vi "CSM - List Status in Broadcast Registry.vi"(8 "error in (no error)":errorcluster) -> (0 "error out":errorcluster, 3 "Status in Registry":string[](array[string]))   [LabVIEW 2020, in "Communicable State Machine.lvlib"]
uses:
  Communicable State Machine.lvlib
  Operation-BroadcastRegistry.ctl
  global-Broadcast Cache Change Flag.vi
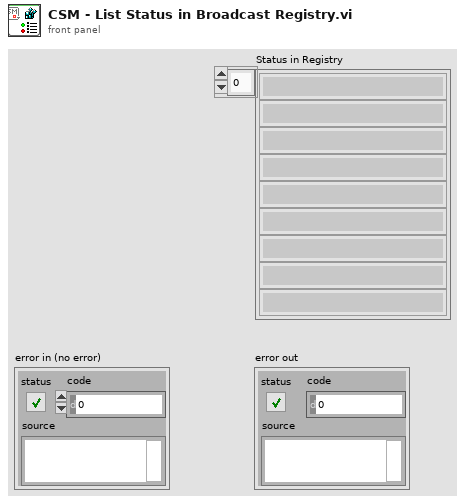
[diagram p1: front panel]
types:
  T1 = typedef "Communicable State Machine.lvlib/Operation-BroadcastRegistry.ctl" = enum16{"Delete Source Module", "Delete Target Module", "Remove Module", "Register", "Unregister", "Check", "List Status", "List Entries"}
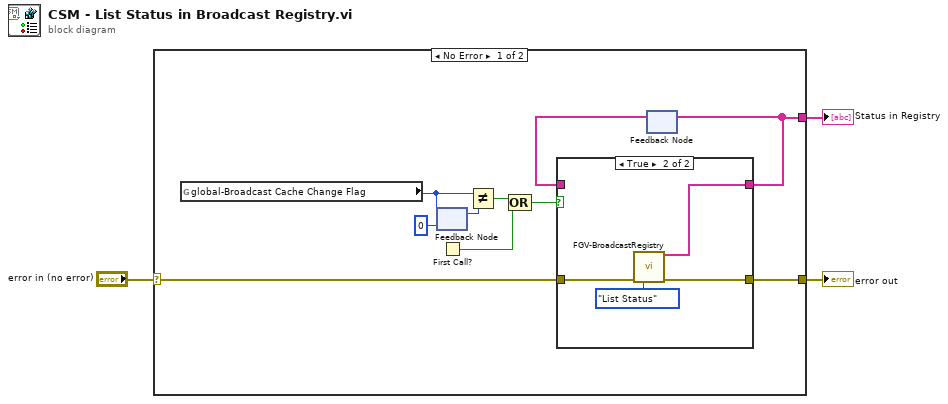
[diagram p0: block diagram]
diagram:
  n1 = case shown="No Error" "error in (no error)" {
    selector: "error in (no error)" -> [w13 w20]
    tunnel: [w6 _] -> w2
    tunnel: [w4 w20] -> w1
    frame No Error {
      n2 = global read "global-Broadcast Cache Change Flag.vi" "global-Broadcast Cache Change Flag"() -> (w10:u64)
      n3 = feedback #1(u64 0 ("global-Broadcast Cache Change Flag")) -> (w11:u64)
      n4 = feedback-in #1(w10) -> ()
      n5 = First Call?() -> (First Call?: T/F=w9:bool)
      n6 = Not Equal?(x=w10, y=w11) -> (x != y?=w8:bool)
      n7 = Compound Arithmetic op=OR(w8, w9) -> (w7:bool)
      n8 = feedback #2() -> (w5:string[])  [unwired: 1 in]
      n9 = case shown="True" w7 {
        tunnel: [w15 w19] -> w4
        tunnel: w13 -> [w15 w18]
        tunnel: [w14 w16] -> w6
        tunnel: w5 -> [w14 _]
        frame False {
        }
        frame True {
          n10 = call "FGV-BroadcastRegistry.vi"("Error in"=w18, "Operation"=Operation-BroadcastRegistry."List Status") -> ("response message"=w16:string[], "Error out"=w19:errorcluster)  [unwired: 12 in]
        }
      }
      n11 = feedback-in #2(w6) -> ()
    }
    frame Error {
    }
  }
  "error out" <- w1
  "Status in Registry" <- w2
